vi "Temperature-Based-Sequential-Control-System.vi"() -> ()   [LabVIEW 2025]
panel:
  out "Temp":dbl
  out "Alarm":bool
  out "Motor":bool
  out "Heater":bool
  in  "Temp":dbl(slide) scale=0.0..1200.0
  in  "Start":bool
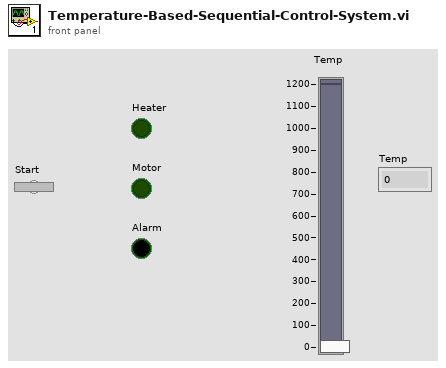
[diagram p1: front panel]
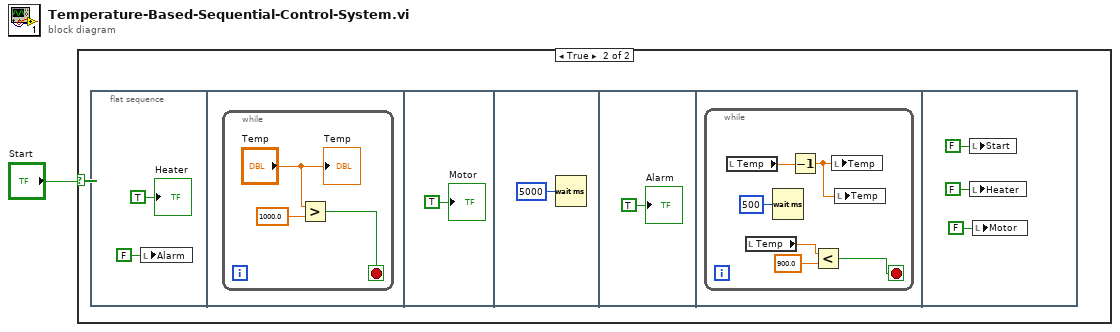
[diagram p0: block diagram]
diagram:
  n1 = case shown="True" "Start" {
    frame False {
    }
    frame True {
      n2 = flat-sequence {
        frame #0 {
          n3 = local write "Alarm"(FALSE ("Alarm")) -> ()
          "Heater" <- TRUE ("Heater")
        }
        frame #1 {
          n4 = while {
            stop <- w4 stop-if-true
            n5 = Greater?(x="Temp", y=1000.0) -> (0:w4:bool)
            "Temp" <- "Temp"
          }
        }
        frame #2 {
          "Motor" <- TRUE ("Motor")
        }
        frame #3 {
          n6 = Wait (ms)(milliseconds to wait=u32 5000) -> ()  [unwired: 1 out]
        }
        frame #4 {
          "Alarm" <- TRUE ("Alarm")
        }
        frame #5 {
          n7 = while {
            stop <- w11 stop-if-true
            n8 = local read "Temp"() -> (w15:dbl)
            n9 = local read "Temp"() -> (w13:dbl)
            n10 = Wait (ms)(milliseconds to wait=u32 500) -> ()  [unwired: 1 out]
            n11 = Decrement(x=w15) -> (x-1=w10:dbl)
            n12 = Less?(x=w13, y=900.0) -> (x < y?=w11:bool)
            n13 = local write "Temp"(w10) -> ()
            n14 = local write "Temp"(w10) -> ()
          }
        }
        frame #6 {
          n15 = local write "Start"(FALSE ("Start")) -> ()
          n16 = local write "Heater"(FALSE ("Heater")) -> ()
          n17 = local write "Motor"(FALSE ("Motor")) -> ()
        }
      }
    }
  }
